vi "CS_cRIO-PB_DP-Master_SlaveInfo.vi"(0 "FPGA VI Reference":T2, 11 "Error":errorcluster) -> (4 "FPGA VI Reference out":T2, 8 "Slave Info List":T1(array[cluster]), 15 "Error out":errorcluster)   [LabVIEW 2013, in "dynamic profibus.lvlib"]
doc: "Returns a list with additional information of the configured DP-Slaves.\n\nFPGA VI Reference:\nReference of the FPGA VI.\n\n\nSlave Info List:\nThe list contains additional information about input and output lengths of the configured DP-Slaves.\n\nFPGA VI Reference out:\nIs a copy of the FPGA VI Reference .\n\nError in:\nPreceding error conditions. If an error has already occurred, the VI returns the value of the error in Error out.\n\nError out:\nError: TRUE if an error occurred.\nStatus: Error code\nInfo: Error description"
uses:
  dynamic profibus.lvlib
  fpga reference.ctl
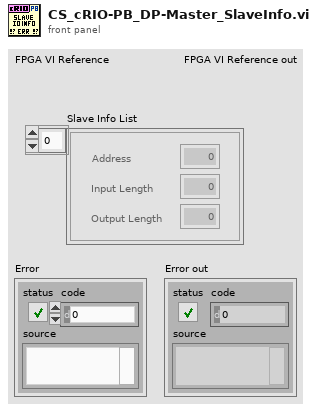
[diagram p1: front panel]
types:
  T1 = cluster{"Address":i8, "Input Length":u8, "Output Length":u8}[]
  T2 = typedef "dynamic profibus.lvlib/fpga reference.ctl" = refnum<k20>
  T3 = enum16{"Start/Stop DP-Master", "Get Input Data", "Set Output Data", "Get Output Data", "Get Diagnostic Data", "Read/Write Data", "Read Diagnostic Data", "Get DPV1 Data", "Set DPV1 Data", "Read/Write DPV1 Data"}
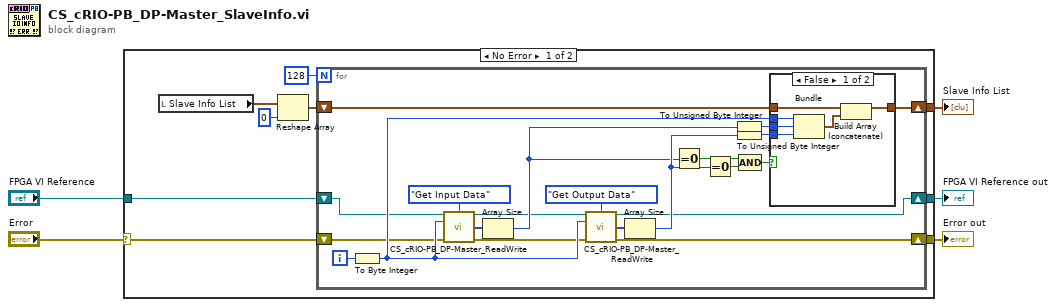
[diagram p0: block diagram]
diagram:
  n1 = case shown="No Error" "Error" {
    selector: "Error" -> [w9 w43]
    tunnel: "FPGA VI Reference" -> [w13 w44]
    tunnel: [w12 _] -> w1
    tunnel: [w8 w43] -> w4
    tunnel: [w7 w44] -> w3
    frame No Error {
      n2 = local read "Slave Info List"() -> (w11:T1)
      n3 = Reshape Array(w11, 0 ("dimension size")) -> (w10:T1)
      n4 = for {
        N: 128 -> [_]
        shift-right: [w20] -> w7
        shift-left: w13 -> [w24]
        shift-right: [w25] -> w8
        shift-left: w9 -> [w27]
        shift-right: [w32] -> w12
        shift-left: w10 -> [w31]
        i -> [w33]
        n5 = To Byte Integer(number=w33) -> (8bit integer=w34:i8)
        n6 = call "CS_cRIO-PB_DP-Master_ReadWrite.vi"("FPGA VI Reference"=w24, "Mode"=T3."Get Input Data", "Slave"=w34, "Error"=w27) -> ("FPGA VI Reference out"=w19:T2, "Data out"=w23:u8[], "Error out"=w26:errorcluster)  [unwired: 8 in, 1 out]
        n7 = Array Size(array=w23) -> (size(s)=w22:i32)
        n8 = call "CS_cRIO-PB_DP-Master_ReadWrite.vi"("FPGA VI Reference"=w19, "Mode"=T3."Get Output Data", "Slave"=w34, "Error"=w26) -> ("FPGA VI Reference out"=w20:T2, "Data out"=w21:u8[], "Error out"=w25:errorcluster)  [unwired: 8 in, 1 out]
        n9 = Array Size(array=w21) -> (size(s)=w35:i32)
        n10 = Equal To 0?(x=w22) -> (x = 0?=w30:bool)
        n11 = Equal To 0?(x=w35) -> (x = 0?=w29:bool)
        n12 = To Unsigned Byte Integer(number=w22) -> (unsigned 8bit integer=w18:u8)
        n13 = To Unsigned Byte Integer(number=w35) -> (unsigned 8bit integer=w17:u8)
        n14 = Compound Arithmetic op=AND(w30, w29) -> (w28:bool)
        n15 = case shown="False" w28 {
          tunnel: [w41 w42] -> w32
          tunnel: w31 -> [w40 w42]
          tunnel: w34 -> [w39 _]
          tunnel: w17 -> [w37 _]
          tunnel: w18 -> [w36 _]
          frame False {
            n16 = Bundle(w39, w36, w37) -> (w38:cluster{i8, u8, u8})  [unwired: 1 in]
            n17 = Build Array (concatenate)(w40, w38) -> (w41:T1)
          }
          frame True {
          }
        }
      }
    }
    frame Error {
    }
  }
  "Error out" <- w4
  "FPGA VI Reference out" <- w3
  "Slave Info List" <- w1
